vi "PH_PP_CurrentMeas.PC read MA DP.vi"(0 "i ref in":refnum<vi>, 5 "error in (no error)":errorcluster) -> (14 "i ref out":refnum<vi>, 19 "error out":errorcluster)   [LabVIEW 2014, in "PH_PP_CurrentMeas.lvlib"]
doc: "This VI reads the relevant RT Clients and sets the data to the GUI (if MA DP is chosen)."
uses:
  PH_PP_CurrentMeas.lvlib
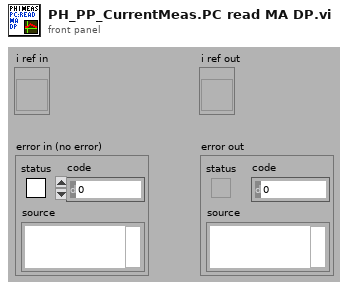
[diagram p1: front panel]
types:
  T1 = typedef "PH_PP_CurrentMeas.lvlib/PH_PP_CurrentMeas.i attribute.ctl" = cluster{"Status":cluster{"GUI Ref Hardware Feedback":refnum<vi>, "Tab Control":refnum<vi>}, "PU 1":cluster{"Instance":string, "Status":T2, "Ref Status ":refnum<vi>, "Data":waveform(dbl)[], "Ref Data":refnum<vi>}, "PU 2":cluster{"Instance":string, "Status":T2, "Ref Status ":refnum<vi>, "Data":waveform(dbl)[], "Ref Data":refnum<vi>}, "PU 3":cluster{"Instance":string, "Status":T2, "Ref Status ":refnum<vi>, "Data":waveform(dbl)[], "Ref Data":refnum<vi>}, "PU 4":cluster{"Instance":string, "Status":T2, "Ref Status ":refnum<vi>, "Data":waveform(dbl)[], "Ref Data":refnum<vi>}, "PU 5":cluster{"Instance":string, "Status":T2, "Ref Status ":refnum<vi>, "Data":waveform(dbl)[], "Ref Data":refnum<vi>}, "FR":cluster{"Instance":string, "Status":T2, "Ref Status ":refnum<vi>, "Data":waveform(dbl)[], "Ref Data":refnum<vi>}, "PA - 19mm 1":cluster{"Instance":string, "Status":T2, "Ref Status ":refnum<vi>}, "PA - 19mm 2":cluster{"Instance":string, "Status":T2, "Ref Status ":refnum<vi>, "no link":bool}, "PA - 45mm":cluster{"Instance":string, "Status":T2, "Ref Status ":refnum<vi>, "no link":bool}, "PA Data":cluster{"Data":waveform(dbl)[], "Ref":refnum<vi>}, "Sequencer":cluster{"Instance":string, "SM State Ref":refnum<vi>}, "Tasks":cluster{"Port":u16, "connection ID":refnum<k5>, "Status":T2, "Ref":refnum<vi>, "Ref Bar":refnum<vi>, "Feedback":cluster{"Received Data Sets":T3[], "Driver Error":errorcluster, "Connection not established":bool, "Error unpacking the data":bool, "No Task defined":bool, "Not triggered yet":bool}, "Data":waveform(dbl)[], "Ref Teststart Task":refnum<vi>}[], "in use":cluster{"MA DP":bool, "FR and PA":bool}, "DAQ Server":string}
  T2 = typedef "PH_StatusHandler.lvlib/PH_StatusHandler.Status.ctl" = i16
  T3 = typedef "PH_PP_CurrentMeas.lvlib/PH_PP_CurrentMeas.CommandCluster.ctl" = cluster{"Command":string, "Data":string, "error out":errorcluster}
  T4 = enum32{"PA 19 DP", "MA 1", "MA 2", "MA 3", "MA 4", "MA 5", "MA FR", "Feedback"}
  T5 = enum32{"PA 19 DP", "MA 1", "MA 2", "MA 3", "MA 4", "MA 5", "MA FR", "Feedback"}[]
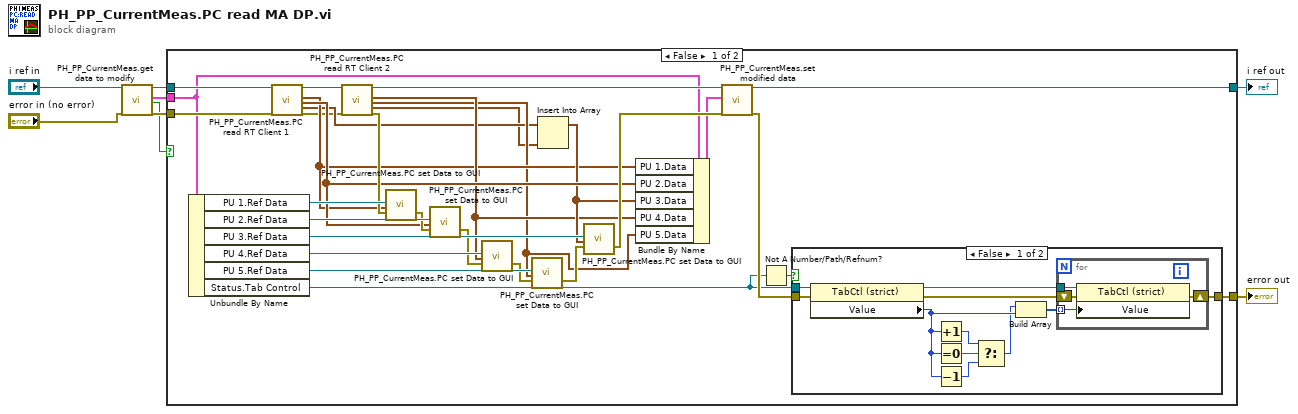
[diagram p0: block diagram]
diagram:
  n1 = call "PH_PP_CurrentMeas.get data to modify.vi"("i ref in"="i ref in", "error in (no error)"="error in (no error)") -> ("i ref out"=w4:refnum<vi>, "i attribute"=w7:T1, "timed out"=w1:bool, "error out"=w6:errorcluster)  [unwired: 14 in]
  n2 = case shown="False" w1 {
    tunnel: [w12 w56] -> w8
    tunnel: w7 -> [w28 _]
    tunnel: w6 -> [w33 w56]
    tunnel: w4 -> [w29 w55]
    tunnel: [w31 w55] -> w2
    frame False {
      n3 = Unbundle By Name(w28) -> ("PU 1.Ref Data"=w34:refnum<vi>, "PU 2.Ref Data"=w35:refnum<vi>, "PU 3.Ref Data"=w38:refnum<vi>, "PU 4.Ref Data"=w36:refnum<vi>, "PU 5.Ref Data"=w37:refnum<vi>, "Status.Tab Control"=w9:refnum<vi>)
      n4 = call "PH_PP_CurrentMeas.PC read RT Client 1.vi"("i ref in"=w29, "error in (no error)"=w33) -> ("i ref out"=w16:refnum<vi>, "Data PU 1"=w18:waveform(dbl)[], "Data PU 2"=w21:waveform(dbl)[], "Data PU 3"=w15:waveform(dbl)[], "error out"=w13:errorcluster)  [unwired: 13 in]
      n5 = call "PH_PP_CurrentMeas.PC read RT Client 2.vi"("i ref in"=w16, "error in (no error)"=w13) -> ("i ref out"=w32:refnum<vi>, "Data PU 4"=w19:waveform(dbl)[], "Data PU 5"=w17:waveform(dbl)[], "Data PU 3"=w14:waveform(dbl)[], "error out"=w23:errorcluster)  [unwired: 13 in]
      n6 = call "PH_PP_CurrentMeas.PC set Data to GUI.vi"("Ref GUI element"=w34, "Data"=w18, "error in (no error)"=w23) -> ("error out"=w26:errorcluster)  [unwired: 16 in]
      n7 = call "PH_PP_CurrentMeas.PC set Data to GUI.vi"("Ref GUI element"=w35, "Data"=w21, "error in (no error)"=w26) -> ("error out"=w22:errorcluster)  [unwired: 16 in]
      n8 = call "PH_PP_CurrentMeas.PC set Data to GUI.vi"("Ref GUI element"=w36, "Data"=w19, "error in (no error)"=w22) -> ("error out"=w25:errorcluster)  [unwired: 16 in]
      n9 = call "PH_PP_CurrentMeas.PC set Data to GUI.vi"("Ref GUI element"=w37, "Data"=w17, "error in (no error)"=w25) -> ("error out"=w24:errorcluster)  [unwired: 16 in]
      n10 = Insert Into Array(array=w15, new element=w14) -> (w20:waveform(dbl)[])  [unwired: 1 in]
      n11 = call "PH_PP_CurrentMeas.PC set Data to GUI.vi"("Ref GUI element"=w38, "Data"=w20, "error in (no error)"=w24) -> ("error out"=w30:errorcluster)  [unwired: 16 in]
      n12 = Bundle By Name(cluster=w28, "PU 1.Data"=w18, "PU 2.Data"=w21, "PU 3.Data"=w20, "PU 4.Data"=w19, "PU 5.Data"=w17) -> (w27:T1)
      n13 = call "PH_PP_CurrentMeas.set modified data.vi"("i ref in"=w32, "i attribute"=w27, "error in (no error)"=w30) -> ("i ref out"=w31:refnum<vi>, "error out"=w11:errorcluster)  [unwired: 15 in]
      n14 = Not A Number/Path/Refnum?(number/path/refnum=w9) -> (NaN/Path/Refnum?=w10:bool)
      n15 = case shown="False" w10 {
        tunnel: [w49 w54] -> w12
        tunnel: w9 -> [w48 _]
        tunnel: w11 -> [w46 w54]
        frame False {
          n16 = property class="TabCtl (strict)"(reference=w48, error in=w46) -> (reference out=w47:refnum<vi>, error out=w45:errorcluster, "Value"=w43:T4)
          n17 = Increment(x=w43) -> (x+1=w41:T4)
          n18 = Equal To 0?(x=w43) -> (x = 0?=w42:bool)
          n19 = Decrement(x=w43) -> (x-1=w40:T4)
          n20 = Select(t=w41, s=w42, f=w40) -> (s? t:f=w39:T4)
          n21 = Build Array(w39, w43) -> (w44:T5)
          n22 = for {
            tunnel: w47 -> [w51]
            shift-right: [w52] -> w49
            shift-left: w45 -> [w53]
            tunnel: w44 -> [w50] mode=indexing
            n23 = property class="TabCtl (strict)"(reference=w51, error in=w53, "Value"=w50) -> (error out=w52:errorcluster)  [unwired: 1 out]
          }
        }
        frame True {
        }
      }
    }
    frame True {
    }
  }
  "error out" <- w8
  "i ref out" <- w2
